vi "setBlockHeader.vi"(1 "Block Timing":T1, 2 "No of Analog. Samples":i32) -> (0 "Output String":string)   [LabVIEW 2013]
uses:
  Controls/blockTiming.ctl
  Globals/measurementGlobal.vi
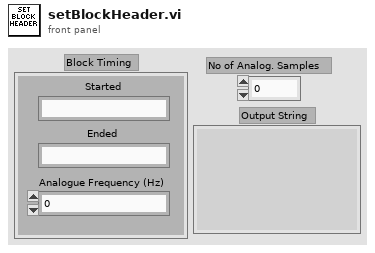
[diagram p1: front panel]
types:
  T1 = typedef "blockTiming.ctl" = cluster{"Started":string, "Ended":string, "Analogue Frequency (Hz)":dbl}
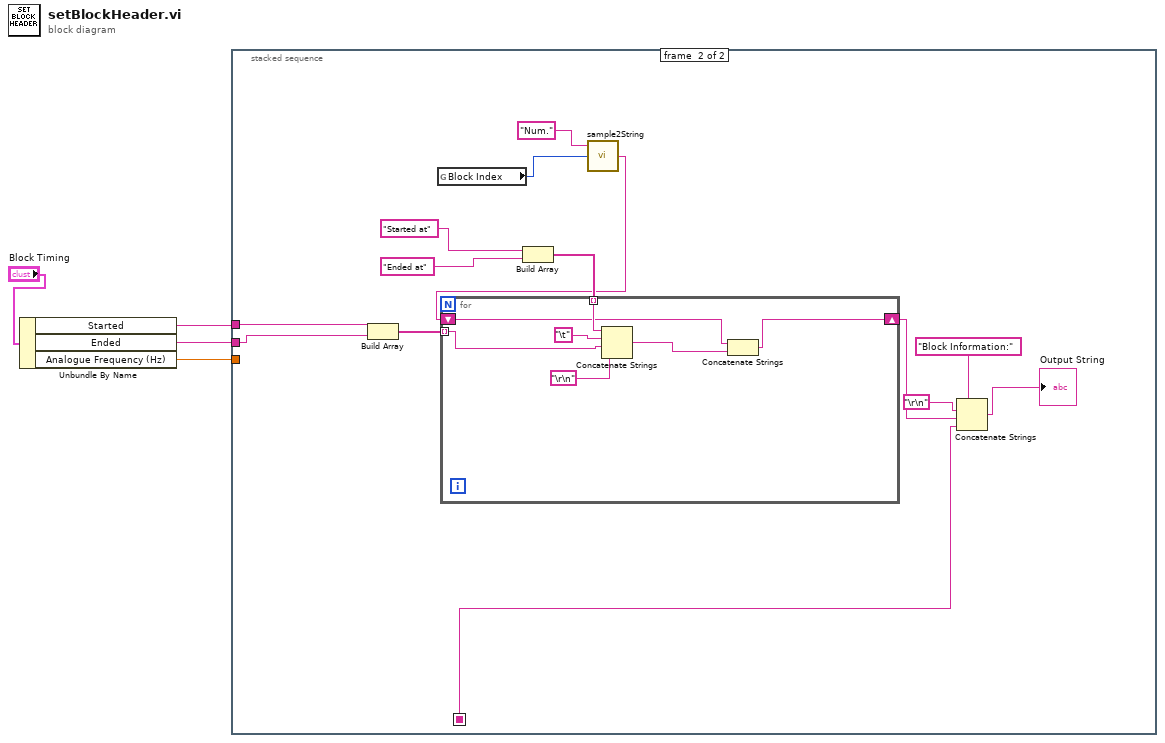
[diagram p0: block diagram]
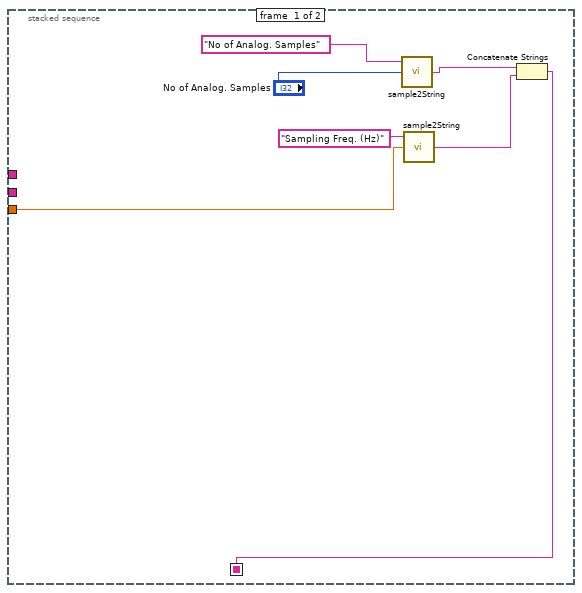
[diagram p2: hidden frame]
diagram:
  n1 = Unbundle By Name("Block Timing") -> ("Started"=w2:string, "Ended"=w1:string, "Analogue Frequency (Hz)"=w3:dbl)
  n2 = stacked-sequence {
    seq-local: [w5 _] -> [_ w14]
    tunnel: w3 -> [w9 _]
    tunnel: w2 -> [_ w21]
    tunnel: w1 -> [_ w20]
    frame #0 {
      n3 = call "sample2String.vi"("Number"="No of Analog. Samples", "Label"="No of Analog. Samples") -> ("Output String"=w8:string)  [unwired: 1 in]
      n4 = call "sample2String.vi"("Number"=w9, "Label"="Sampling Freq. (Hz)") -> ("Output String"=w7:string)  [unwired: 1 in]
      n5 = Concatenate Strings(w8, w7) -> (w5:string)
    }
    frame #1 {
      n6 = Build Array(w21, w20) -> (w19:string[])
      n7 = global read "measurementGlobal.vi" "Block Index"() -> (w24:i32)
      n8 = Build Array("Started at", "Ended at") -> (w18:string[])
      n9 = call "sample2String.vi"("Number"=w24, "Label"="Num.") -> ("Output String"=w17:string)  [unwired: 1 in]
      n10 = for {
        tunnel: w19 -> [w26] mode=indexing
        tunnel: w18 -> [w32] mode=indexing
        shift-right: [w27] -> w15
        shift-left: w17 -> [w29]
        n11 = Concatenate Strings(w32, "\t", w26, "\r\n") -> (w28:string)
        n12 = Concatenate Strings(w29, w28) -> (w27:string)
      }
      n13 = Concatenate Strings("Block Information:" ("string"), "\r\n", w15, w14) -> (→"Output String":string)
    }
  }
